vi "Initialize.vi"(8 "error in (no error)":errorcluster, 11 "Serial in":refnum<class "Serial.lvclass">) -> (0 "error out":errorcluster, 3 "MB_TCP out":refnum<class "Serial.lvclass">)   [LabVIEW 2021, in "Serial.lvclass"]
uses:
  Serial.lvclass
  Serial.lvclass/Serial.ctl
  MB Param/MBTCP Param/MBTCP Param.lvclass
  MB/ctl/MB timeouts.ctl
  MB/Modbus Master CR.lvclass
  Transmission Data Unit/Transmission Data Unit.lvclass
  Transmission Data Unit/RTU/RTU Data Unit.lvclass
  Transmission Data Unit/ASCII/ASCII Data Unit.lvclass
  C:/my_projects/projects/Algorithms/Labview/21/Modbus_v121c/Network Protocol/MB/Modbus Master CR.lvclass
  C:/my_projects/projects/Algorithms/Labview/21/Modbus_v121c/Network Protocol/Network Master/Network Master.lvclass
  C:/my_projects/projects/Algorithms/Labview/21/Modbus_v121c/Network Protocol/Network Protocol.lvclass
  C:/my_projects/projects/Algorithms/Labview/21/Modbus_v121c/Network Protocol/M7000/Serial/Serial.lvclass
  Transmission Data Unit/Serial Interface/Serial Data Unit.lvclass
  C:/my_projects/projects/Algorithms/Labview/21/Modbus_v121c/Transmission Data Unit/Transmission Data Unit.lvclass
  C:/my_projects/projects/Algorithms/Labview/21/Modbus_v121c/Transmission Data Unit/Serial Interface/Serial Data Unit.lvclass
  Network Master/Network Master.lvclass
  C:/my_projects/projects/Algorithms/Labview/21/Modbus_v121c/Transmission Data Unit/RTU/RTU Data Unit.lvclass
  C:/my_projects/projects/Algorithms/Labview/21/Modbus_v121c/Transmission Data Unit/ASCII/ASCII Data Unit.lvclass
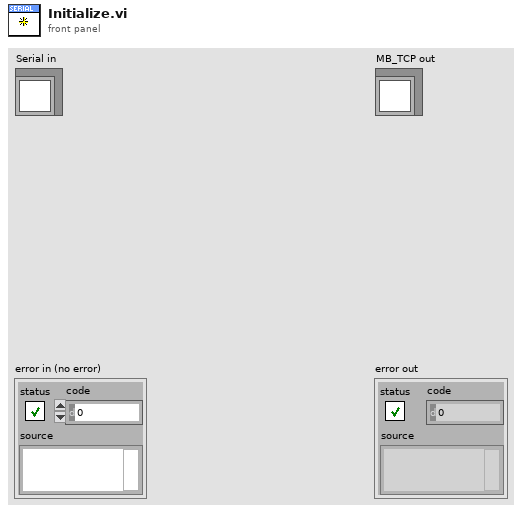
[diagram p1: front panel]
types:
  T1 = typedef "Modbus Master CR.lvclass/MB timeouts.ctl" = cluster{"reconn_timeout":i32, "N attempt max":i32, "t_reset_TTL":i32, "period":i32}
  T2 = typedef "MBParam.lvlib/MBTCP Param.lvclass/timeouts.ctl" = cluster{"conn_timeout":i32, "reconn_timeout":i32, "N attempt max":i32, "t_reset_TTL":i32, "write_timeout":i32, "read_timeout":i32, "period":i32}
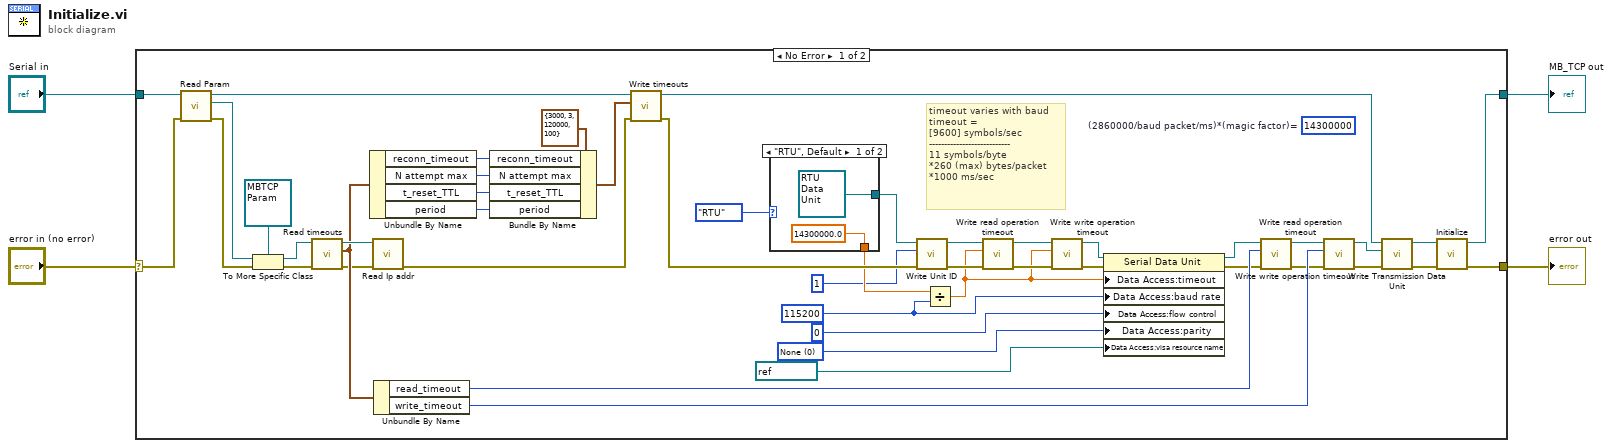
[diagram p0: block diagram]
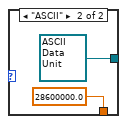
[diagram p2: hidden frame]
diagram:
  n1 = case shown="No Error" "error in (no error)" {
    selector: "error in (no error)" -> [w42 w56]
    tunnel: [w32 w56] -> w1
    tunnel: [w33 w57] -> w2
    tunnel: "Serial in" -> [w39 w57]
    frame No Error {
      w17 = u16 0 items=["None", "Odd", "Even"] ("parity (Even)")
      w11 = u32 115200 ("baud rate (9600)")
      (unwired) u32 14300000  # (2860000/baud packet/ms)*(magic factor)=
      # "timeout varies with baud\ntimeout =\n[9600] symbols/sec\n---------------------------\n11 symbols/byte\n*260 (max) bytes/packet\n*1000 ms/sec"
      n2 = call "Read Param.vi"("error in (no error)"=w42, "MB_TCP in"=w39) -> ("error out"=w41:errorcluster, "Param"=w38:refnum<class "MB Param.lvclass">, "MB_TCP out"=w37:refnum<class "Serial.lvclass">)  [unwired: 7 in]
      n3 = To More Specific Class(target class=refnum<class "MBTCP Param.lvclass"> refnum ("MBParam.lvlib:MBTCP Param.lvclass"), reference=w38, error in=w41) -> (specific class reference=w40:refnum<class "MBTCP Param.lvclass">, error out=w50:errorcluster)
      n4 = call "Read timeouts.vi"("error in (no error)"=w50, "MBParam in"=w40) -> ("error out"=w35:errorcluster, "timeouts"=w36:T2, "MBParam out"=w43:refnum<class "MBTCP Param.lvclass">)  [unwired: 7 in]
      n5 = Unbundle By Name(w36) -> ("reconn_timeout"=w48:i32, "N attempt max"=w45:i32, "t_reset_TTL"=w46:i32, "period"=w47:i32)
      n6 = call "Read Ip addr.vi"("error in (no error)"=w35, "MBParam in"=w43) -> ("error out"=w34:errorcluster)  [unwired: 7 in, 2 out]
      n7 = Unbundle By Name(w36) -> ("read_timeout"=w30:i32, "write_timeout"=w29:i32)
      n8 = Bundle By Name(cluster=T1 {"reconn_timeout"=3000, "N attempt max"=3, "t_reset_TTL"=120000, "period"=100} ("MB timeouts"), "reconn_timeout"=w48, "N attempt max"=w45, "t_reset_TTL"=w46, "period"=w47) -> (w44:T1)
      n9 = call "Write timeouts.vi"("error in (no error)"=w34, "MB timeouts"=w44, "MB_TCP in"=w37) -> ("error out"=w31:errorcluster, "MB_TCP out"=w6:refnum<class "Serial.lvclass">)  [unwired: 7 in]
      n10 = case shown="\"RTU\", Default" enum16{"RTU", "ASCII"}."RTU" ("serial type") {
        tunnel: [refnum<class "RTU Data Unit.lvclass"> refnum ("RTU Data Unit") refnum<class "ASCII Data Unit.lvclass"> refnum ("ASCII Data Unit")] -> w26
        tunnel: [14300000.0 ("x") 28600000.0 ("x")] -> w21
        frame "RTU", Default {
        }
        frame "ASCII" {
        }
      }
      n11 = call "Write Unit ID.vi"("error in"=w31, "unit ID"=u8 1, "transmission data unit in"=w26) -> ("error out"=w22:errorcluster, "transmission data unit out"=w25:refnum<class "Serial Data Unit.lvclass">)  [unwired: 7 in]
      n12 = Divide(x=w21, y=w11) -> (x/y=w20:dbl)
      n13 = call "Write read operation timeout.vi"("error in (no error)"=w22, "read operation timeout"=w20, "transmission data unit in"=w25) -> ("error out"=w23:errorcluster, "transmission data unit out"=w24:refnum<class "Serial Data Unit.lvclass">)  [unwired: 7 in]
      n14 = call "Write write operation timeout.vi"("error in (no error)"=w23, "write operation timeout"=w20, "transmission data unit in"=w24) -> ("error out"=w12:errorcluster, "transmission data unit out"=w10:refnum<class "Serial Data Unit.lvclass">)  [unwired: 7 in]
      n15 = property class="Serial Data Unit"(reference=w10, error in=w12, "Data Access:timeout"=w20, "Data Access:baud rate"=w11, "Data Access:flow control"=u16 0 ("Flow Control"), "Data Access:parity"=w17, "Data Access:visa resource name"=refnum<visa-resource-name> "COM1" ("VISA resource name")) -> (reference out=w8:refnum<class "Serial Data Unit.lvclass">, error out=w9:errorcluster)
      n16 = call "Write read operation timeout.vi"("error in (no error)"=w9, "read operation timeout"=w30, "transmission data unit in"=w8) -> ("error out"=w27:errorcluster, "transmission data unit out"=w28:refnum<class "Serial Data Unit.lvclass">)  [unwired: 7 in]
      n17 = call "Write write operation timeout.vi"("error in (no error)"=w27, "write operation timeout"=w29, "transmission data unit in"=w28) -> ("error out"=w13:errorcluster, "transmission data unit out"=w14:refnum<class "Serial Data Unit.lvclass">)  [unwired: 7 in]
      n18 = call "Write Transmission Data Unit.vi"("error in (no error)"=w13, "Transmission Data Unit"=w14, "Network Master in"=w6) -> ("error out"=w7:errorcluster, "Network Master out"=w5:refnum<class "Serial.lvclass">)  [unwired: 7 in]
      n19 = call-parent "Initialize.vi"("error in (no error)"=w7, "MB in"=w5) -> ("error out"=w32:errorcluster, "MB out"=w33:refnum<class "Serial.lvclass">)  [unwired: 8 in]
    }
    frame Error {
    }
  }
  "error out" <- w1
  "MB_TCP out" <- w2
